vi "Stop Core.vi"(10 "final error code":i32, 11 "Guardar Tipo CSV in":refnum<class "Guardar Tipo CSV.lvclass">) -> (3 "Guardar Tipo CSV out":refnum<class "Guardar Tipo CSV.lvclass">)   [LabVIEW 2020, in "Guardar Tipo CSV.lvlib" / "Guardar Tipo CSV.lvclass"]
doc: "(<B>Filename</B>: Actor Framework.lvlib:Actor.lvclass:Stop Core.vi)\n\nDefines what the actor does before it stops. Use the <B>final error code</B> input to determine whether the actor shut down in response to an error.\n\nBy default, this method passes the Stop message along to all auto-stop nested actors. A descendant class may override this method to define additional behavior, such as shutting down any processes the actor initiated in its override of the Actor Core method."
uses:
  Guardar Tipo CSV.lvclass
  <vilib>/ActorFramework/Actor/Actor.lvclass
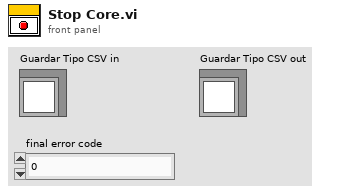
[diagram p1: front panel]
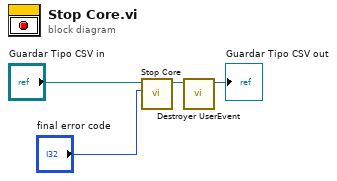
[diagram p0: block diagram]
diagram:
  n1 = call-parent "Stop Core.vi"("final error code"="final error code", "Actor in"="Guardar Tipo CSV in") -> ("Actor out"=w2:refnum<class "Guardar Tipo CSV.lvclass">)  [unwired: 9 in]
  n2 = call "Destroyer UserEvent.vi"("Guardar Tipo CSV in"=w2) -> ("Guardar Tipo CSV out"=→"Guardar Tipo CSV out":refnum<class "Guardar Tipo CSV.lvclass">)  [unwired: 9 in, 1 out]
